vi "Get_time.vi"() -> (3 "Elapsed Time (s)":dbl)   [LabVIEW 2013]
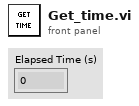
[diagram p1: front panel]
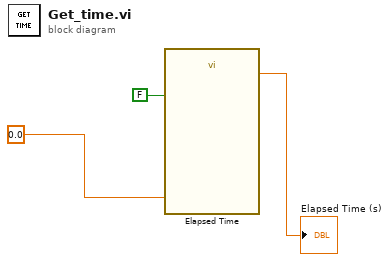
[diagram p0: block diagram]
diagram:
  n1 = call "Elapsed Time"("Auto Reset"=FALSE, "Set Start Time (s)"=0.0) -> ("Elapsed Time (s)"=→"Elapsed Time (s)":dbl)  [unwired: 10 in, 7 out]
